vi "hist.vi"() -> ()   [LabVIEW 2014]
uses:
  <instrlib>/Agilent 532XX Series/Public/Configure/Configure Channel (Basic).vi
  <instrlib>/Agilent 532XX Series/Public/Configure/Configure Channel (Voltage Range).vi
  <instrlib>/Agilent 532XX Series/Public/Configure/Configure Channel (Slop).vi
  <instrlib>/Agilent 532XX Series/Public/Configure/Configure Channel (Threshold Voltage).vi
  <instrlib>/Agilent 532XX Series/Public/Configure/Measurement/Configure Measurement (Time Interval).vi
  <instrlib>/Agilent 532XX Series/Public/Data/Read Measurement (Multiple).vi
  <instrlib>/Agilent 532XX Series/Agilent 532XX Series.lvlib
  <vilib>/Analysis/NI_AALBase.lvlib
panel:
  out "Histogram Graph":T1(graph)
  out "Measurements":dbl[](array[numeric]) format="%#_12g"
  out "error out":errorcluster
  in  "VISA resource name":refnum<visa-resource-name>
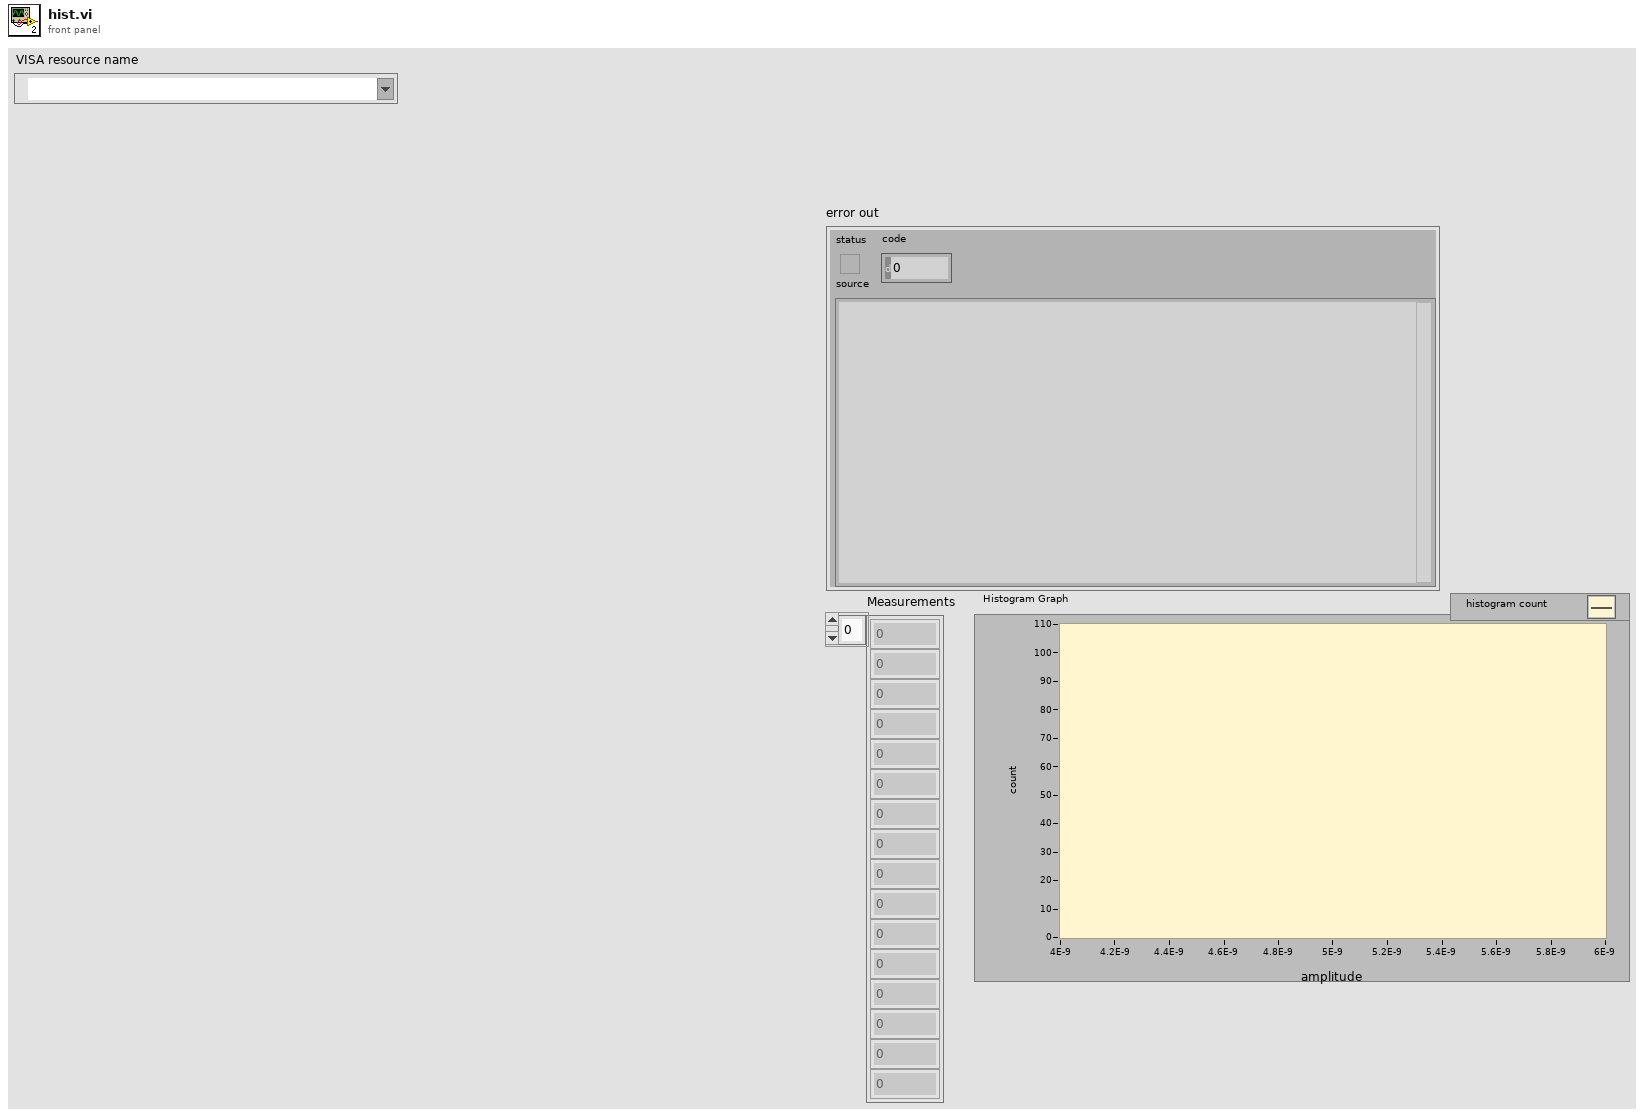
[diagram p1: front panel]
types:
  T1 = cluster{"X Values":dbl[], "Histogram: h(x)":i32[]}
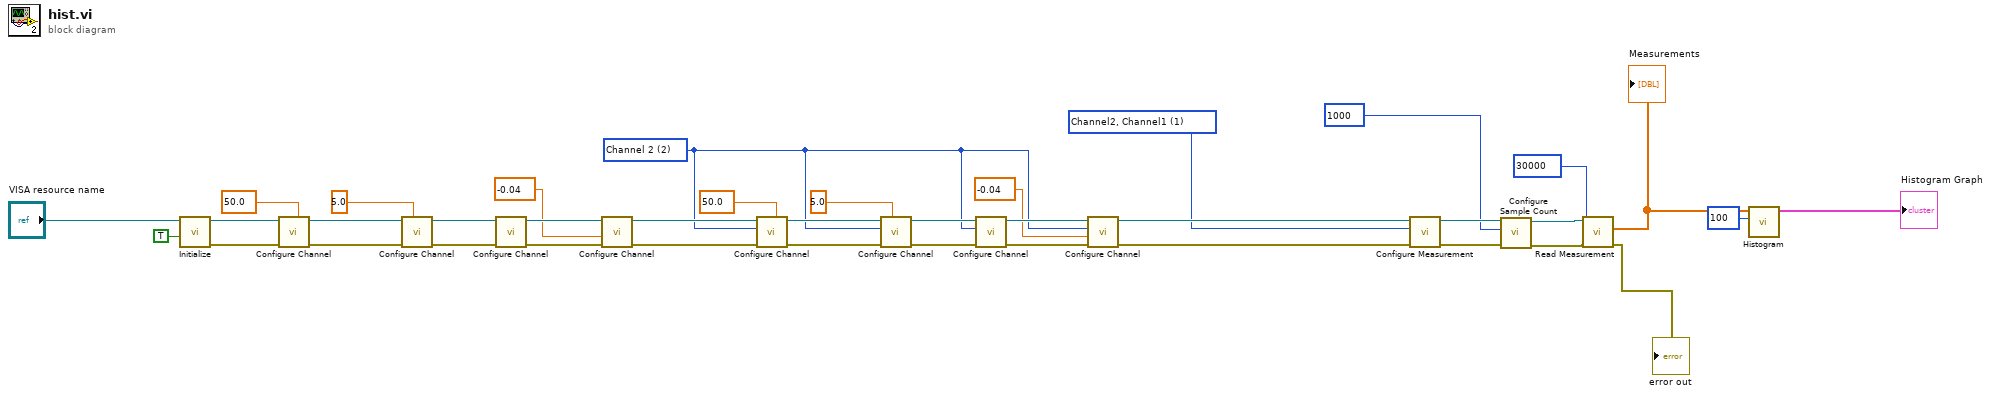
[diagram p0: block diagram]
diagram:
  w11 = 1 items=["Channel1, Channel2", "Channel2, Channel1", " Channel1", "Channel2"] ("Measurement Channels (0: Channel1, Channel2)")
  w14 = 2 items=["Channel 1"=1, "Channel 2"=2] ("Channel (1: Channel 1)")
  w25 = 50.0 items=["50"=50.0, "1E+6"=1000000.0] ("Impedance (1E+6 Ohm)")
  w34 = 50.0 items=["50"=50.0, "1E+6"=1000000.0] ("Impedance (1E+6 Ohm)")
  n1 = call <instrlib>:"Initialize.vi"("Reset (True)"=TRUE, "VISA resource name"="VISA resource name") -> ("error out"=w36:errorcluster, "VISA resource name out"=w35:refnum<visa-resource-name>)  [unwired: 8 in]
  n2 = call-poly <instrlib>:"Configure Channel.vi"("Impedance (1E+6 Ohm)"=w34, "error in (no error)"=w36, "VISA resource name"=w35) -> ("error out"=w31:errorcluster, "VISA resource name out"=w32:refnum<visa-resource-name>)  [unwired: 7 in]
  n3 = call-poly <instrlib>:"Configure Channel.vi"("Voltage Range (5V)"=5.0, "error in (no error)"=w31, "VISA resource name"=w32) -> ("error out"=w29:errorcluster, "VISA resource name out"=w30:refnum<visa-resource-name>)  [unwired: 7 in]
  n4 = call-poly <instrlib>:"Configure Channel.vi"("error in (no error)"=w29, "VISA resource name"=w30) -> ("error out"=w28:errorcluster, "VISA resource name out"=w27:refnum<visa-resource-name>)  [unwired: 8 in]
  n5 = call-poly <instrlib>:"Configure Channel.vi"("error in (no error)"=w28, "Threshold Voltage (0 V)"=-0.04, "VISA resource name"=w27) -> ("error out"=w15:errorcluster, "VISA resource name out"=w16:refnum<visa-resource-name>)  [unwired: 7 in]
  n6 = call-poly <instrlib>:"Configure Channel.vi"("Impedance (1E+6 Ohm)"=w25, "error in (no error)"=w15, "Channel (1: Channel 1)"=w14, "VISA resource name"=w16) -> ("error out"=w22:errorcluster, "VISA resource name out"=w23:refnum<visa-resource-name>)  [unwired: 6 in]
  n7 = call-poly <instrlib>:"Configure Channel.vi"("Voltage Range (5V)"=5.0, "error in (no error)"=w22, "Channel (1: Channel 1)"=w14, "VISA resource name"=w23) -> ("error out"=w20:errorcluster, "VISA resource name out"=w21:refnum<visa-resource-name>)  [unwired: 6 in]
  n8 = call-poly <instrlib>:"Configure Channel.vi"("error in (no error)"=w20, "Channel (1: Channel 1)"=w14, "VISA resource name"=w21) -> ("error out"=w19:errorcluster, "VISA resource name out"=w18:refnum<visa-resource-name>)  [unwired: 7 in]
  n9 = call-poly <instrlib>:"Configure Channel.vi"("error in (no error)"=w19, "Threshold Voltage (0 V)"=-0.04, "Channel (1: Channel 1)"=w14, "VISA resource name"=w18) -> ("error out"=w13:errorcluster, "VISA resource name out"=w12:refnum<visa-resource-name>)  [unwired: 6 in]
  n10 = call-poly <instrlib>:"Configure Measurement.vi"("error in (no error)"=w13, "Measurement Channels (0: Channel1, Channel2)"=w11, "VISA resource name"=w12) -> ("error out"=w9:errorcluster, "VISA resource name out"=w10:refnum<visa-resource-name>)  [unwired: 7 in]
  n11 = call <instrlib>:"Configure Sample Count.vi"("error in (no error)"=w9, "Sample Count (1)"=1000, "VISA resource name"=w10) -> ("error out"=w5:errorcluster, "VISA resource name out"=w6:refnum<visa-resource-name>)  [unwired: 7 in]
  n12 = call-poly <instrlib>:"Read Measurement.vi"("error in (no error)"=w5, "Timeout (10000 ms)"=u32 30000, "VISA resource name"=w6) -> ("error out"=→"error out":errorcluster, "Measurements"=w4:dbl[])  [unwired: 6 in, 1 out]
  "Measurements" <- w4
  n13 = call <vilib>:"Histogram.vi"("intervals"=100, "X"=w4) -> ("Histogram Graph"=→"Histogram Graph":T1)  [unwired: 6 in, 3 out]
